vi "ReadPhysicalChannel.vi"(8 "error in (no error)":errorcluster, 11 "DataVer2 in":refnum<class "DataVer2.lvclass">) -> (0 "error out":errorcluster, 2 "PhysicalChannel":string, 3 "DataVer2 out":refnum<class "DataVer2.lvclass">)   [LabVIEW 2013, in "DataVer2.lvclass"]
uses:
  DataVer2.lvclass
  DataVer2.lvclass/DataVer2.ctl
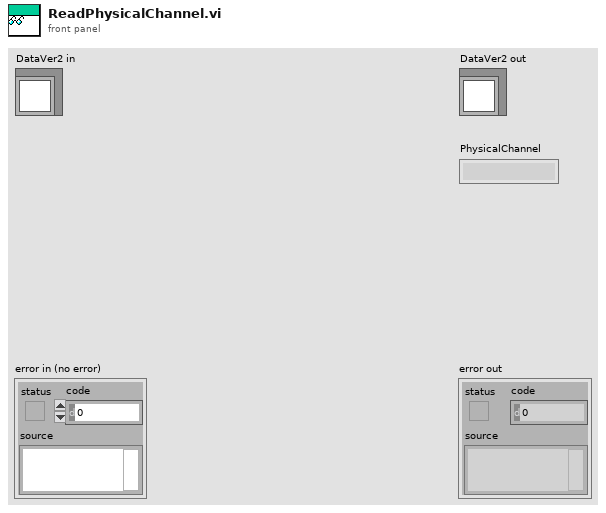
[diagram p1: front panel]
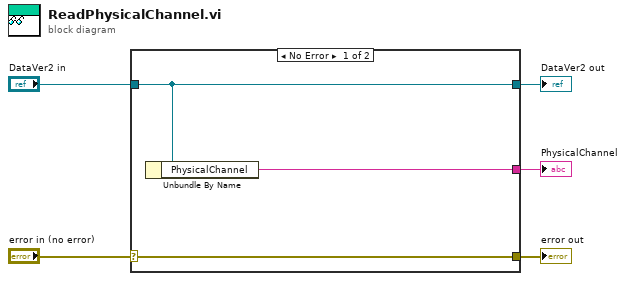
[diagram p0: block diagram]
diagram:
  n1 = case shown="No Error" "error in (no error)" {
    selector: "error in (no error)" -> [w8 w9]
    tunnel: [w8 w9] -> w4
    tunnel: [w7 w10] -> w2
    tunnel: "DataVer2 in" -> [w7 w10]
    tunnel: [w6 _] -> w1
    frame No Error {
      n2 = Unbundle By Name(w7) -> ("PhysicalChannel"=w6:string)
    }
    frame Error {
    }
  }
  "error out" <- w4
  "DataVer2 out" <- w2
  "PhysicalChannel" <- w1
